vi "Start Functional Test.vi"(5 "New Status of Positions":bool[](array[boolean]), 7 "Rack Number":i16=1 min=1 max=16, 11 "System#":u8=1 min=1 max=16) -> ()   [LabVIEW 2021]
uses:
  Main Controls System v8.0/AutoAge Globals.vi
panel:
  out "At least 1 position\nhas started":bool
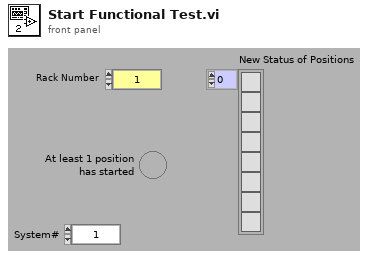
[diagram p1: front panel]
types:
  T1 = enum16{"open", "replace", "create", "open or create", "replace or create", "replace or create with confirmation"}
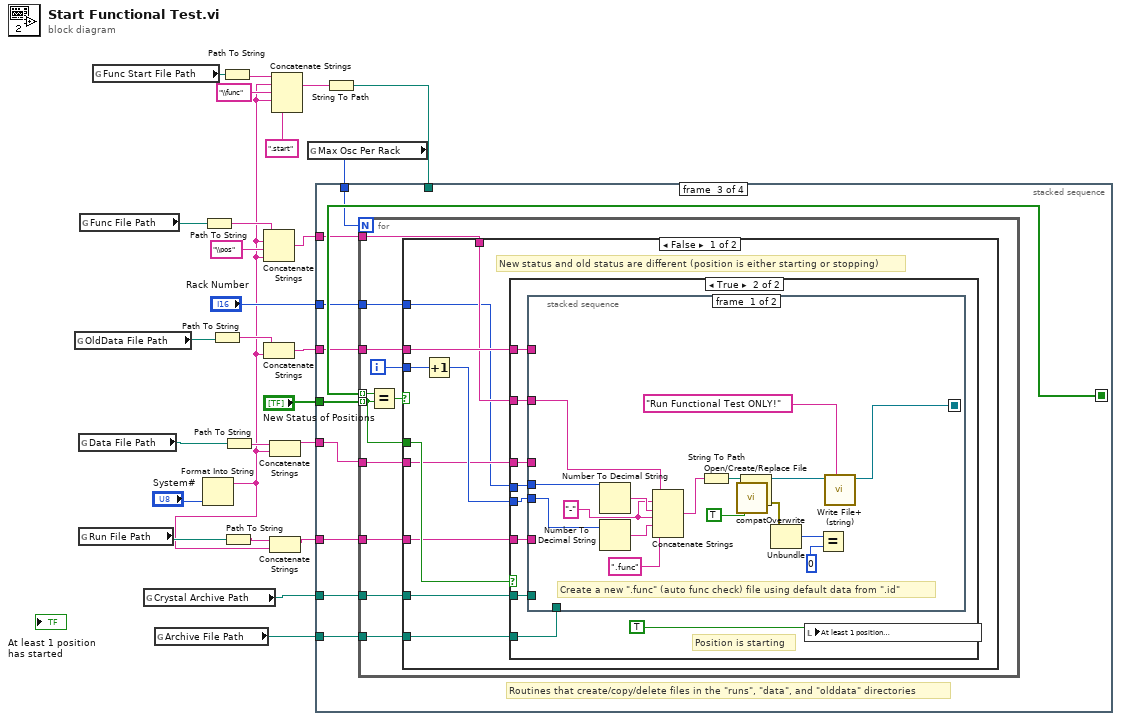
[diagram p0: block diagram]
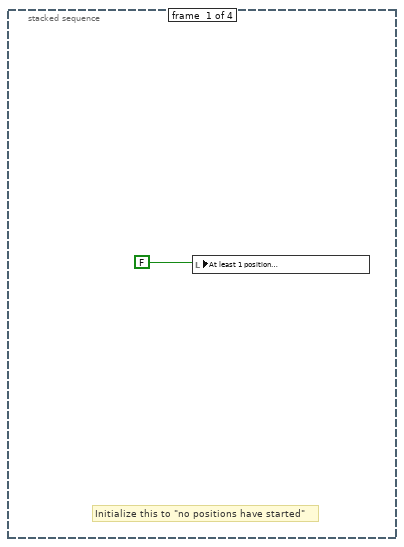
[diagram p2: hidden frame]
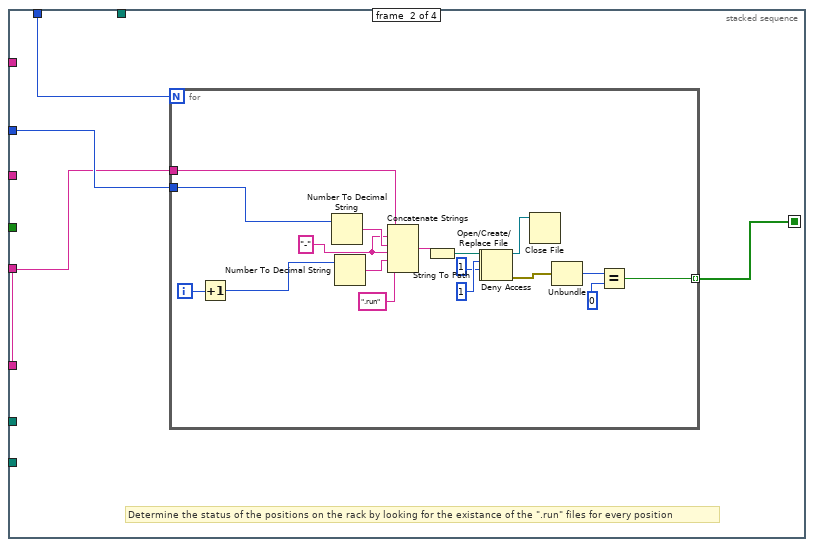
[diagram p3: hidden frame]
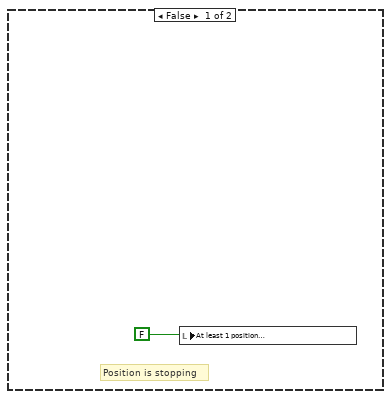
[diagram p4: hidden frame]
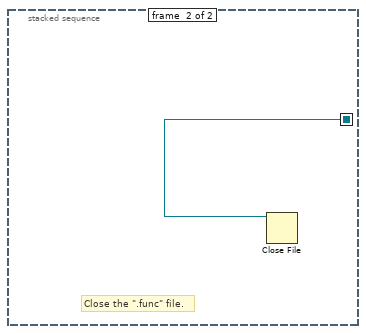
[diagram p5: hidden frame]
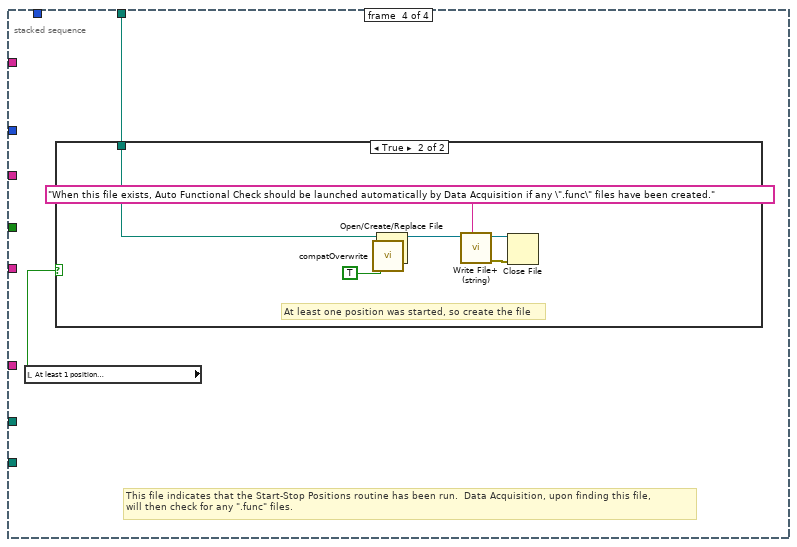
[diagram p7: hidden frame]
diagram:
  n1 = global read "AutoAge Globals.vi" "OldData File Path"() -> (w12:path)
  n2 = global read "AutoAge Globals.vi" "Data File Path"() -> (w11:path)
  n3 = global read "AutoAge Globals.vi" "Run File Path"() -> (w10:path)
  n4 = global read "AutoAge Globals.vi" "Func File Path"() -> (w13:path)
  n5 = global read "AutoAge Globals.vi" "Func Start File Path"() -> (w14:path)
  n6 = global read "AutoAge Globals.vi" "Crystal Archive Path"() -> (w9:path)
  n7 = global read "AutoAge Globals.vi" "Archive File Path"() -> (w8:path)
  n8 = Format Into String("System#") -> (resulting string=w2:string)  [unwired: 3 in, 1 out]
  n9 = Path To String(path=w13) -> (string=w18:string)
  n10 = Path To String(path=w12) -> (string=w20:string)
  n11 = Path To String(path=w14) -> (string=w6:string)
  n12 = Path To String(path=w10) -> (string=w21:string)
  n13 = Path To String(path=w11) -> (string=w24:string)
  n14 = Concatenate Strings(w18, w2, "\\pos" ("Substring"), w2) -> (w17:string)
  n15 = Concatenate Strings(w20, w2) -> (w19:string)
  n16 = Concatenate Strings(w24, w2) -> (w23:string)
  n17 = Concatenate Strings(w21, w2) -> (w22:string)
  n18 = Concatenate Strings(w6, w2, "\\func" ("Substring"), w2, ".start" ("Substring")) -> (w16:string)
  n19 = global read "AutoAge Globals.vi" "Max Osc Per Rack"() -> (w1:u16)
  n20 = String To Path(string=w16) -> (path=w15:path)
  n21 = stacked-sequence {
    seq-local: [_ w30 _ _] -> [_ _ w60 _]
    tunnel: "Rack Number" -> [_ w31 w51 _]
    tunnel: "New Status of Positions" -> [_ _ w59 _]
    tunnel: w22 -> [_ w29 w56 _]
    tunnel: w23 -> [_ _ w57 _]
    tunnel: w19 -> [_ _ w55 _]
    tunnel: w8 -> [_ _ w54 _]
    tunnel: w9 -> [_ _ w53 _]
    tunnel: w17 -> [_ _ w52 _]
    tunnel: w15 -> [_ _ _ w110]
    tunnel: w1 -> [_ w28 w58 _]
    frame #0 {
      # "Initialize this to \"no positions have started\""
      n22 = local write "At least 1 position\nhas started"(FALSE) -> ()
    }
    frame #1 {
      # "Determine the status of the positions on the rack by looking for the existance of the \".run\" files for every position"
      n23 = for {
        N: w28 -> [_]
        tunnel: [w49] -> w30 mode=indexing
        tunnel: w31 -> [w39]
        tunnel: w29 -> [w34]
        i -> [w50]
        w35 = "-"
        n24 = Increment(x=w50) -> (x+1=w36:i32)
        n25 = Number To Decimal String(number=w39) -> (decimal integer string=w38:string)  [unwired: 1 in]
        n26 = Number To Decimal String(number=w36) -> (decimal integer string=w37:string)  [unwired: 1 in]
        n27 = Concatenate Strings(w34, w35, w38, w35, w37, ".run") -> (w48:string)
        n28 = String To Path(string=w48) -> (path=w47:path)
        n29 = Open/Create/Replace File(file path (use dialog)=w47, access (0:read/write)=1) -> (refnum out=w32:refnum<file>, error out=w33:errorcluster)  [unwired: 4 in, 1 out]
        n30 = Deny Access(4:w33, 6:1, 7:w32) -> (0:w44:errorcluster, 3:w41:refnum<file>)
        n31 = Close File(refnum=w41) -> ()  [unwired: 1 in, 2 out]
        n32 = Unbundle(w44) -> ("code"=w42:i32)  [unwired: 2 out]
        n33 = Equal?(x=w42, y=0) -> (x = y?=w49:bool)
      }
    }
    frame #2 {
      # "Routines that create/copy/delete files in the \"runs\", \"data\", and \"olddata\" directories"
      n34 = for {
        N: w58 -> [_]
        tunnel: w60 -> [w70] mode=indexing
        tunnel: w59 -> [w69] mode=indexing
        tunnel: w57 -> [w67]
        tunnel: w56 -> [w66]
        tunnel: w55 -> [w65]
        tunnel: w54 -> [w64]
        tunnel: w53 -> [w63]
        tunnel: w52 -> [w62]
        tunnel: w51 -> [w61]
        i -> [w68]
        n35 = Equal?(x=w70, y=w69) -> (x = y?=w71:bool)
        n36 = case shown="False" w71 {
          tunnel: w69 -> [w81 _]
          tunnel: w68 -> [w80 _]
          tunnel: w67 -> [w78 _]
          tunnel: w66 -> [w77 _]
          tunnel: w65 -> [w76 _]
          tunnel: w64 -> [w75 _]
          tunnel: w63 -> [w74 _]
          tunnel: w62 -> [w73 _]
          tunnel: w61 -> [w72 _]
          frame False {
            # "New status and old status are different (position is either starting or stopping)"
            n37 = Increment(x=w80) -> (x+1=w79:i32)
            n38 = case shown="True" w81 {
              tunnel: w72 -> [_ w83]
              tunnel: w79 -> [_ w91]
              tunnel: w78 -> [_ w89]
              tunnel: w77 -> [_ w85]
              tunnel: w76 -> [_ w88]
              tunnel: w75 -> [_ w87]
              tunnel: w74 -> [_ w86]
              tunnel: w73 -> [_ w84]
              frame False {
                # "Position is stopping"
                n39 = local write "At least 1 position\nhas started"(FALSE) -> ()
              }
              frame True {
                # "Position is starting"
                n40 = stacked-sequence {
                  seq-local: [w96 _] -> [_ w109]
                  tunnel: w83 -> [w97 _]
                  tunnel: w91 -> [w98 _]
                  tunnel: w89 -> [_ _]
                  tunnel: w88 -> [_ _]
                  tunnel: w87 -> [_ _]
                  tunnel: w86 -> [_ _]
                  tunnel: w85 -> [_ _]
                  tunnel: w84 -> [w94 _]
                  frame #0 {
                    w95 = "-"
                    # "Create a new \".func\" (auto func check) file using default data from \".id\""
                    n41 = Number To Decimal String(number=w97) -> (decimal integer string=w101:string)  [unwired: 1 in]
                    n42 = Number To Decimal String(number=w98) -> (decimal integer string=w100:string)  [unwired: 1 in]
                    n43 = Concatenate Strings(w94, w95, w101, w95, w100, ".func") -> (w99:string)
                    n44 = String To Path(string=w99) -> (path=w107:path)
                    n45 = call <vilib>:"compatOverwrite.vi"("overwrite (F)"=TRUE) -> ("overwrite?"=w92:T1)
                    n46 = Open/Create/Replace File(file path (use dialog)=w107, operation (0:open)=w92) -> (refnum out=w103:refnum<file>, error out=w106:errorcluster)  [unwired: 4 in, 1 out]
                    n47 = Unbundle(w106) -> ("code"=w105:i32)  [unwired: 2 out]
                    n48 = Equal?(x=w105, y=0) -> ()  [unwired: 1 out]
                    n49 = call <vilib>:"Write File+ (string).vi"("string"="Run Functional Test ONLY!", "refnum"=w103) -> ("dup refnum"=w96:refnum<file>)  [unwired: 5 in, 2 out]
                  }
                  frame #1 {
                    # "Close the \".func\" file."
                    n50 = Close File(refnum=w109) -> ()  [unwired: 1 in, 2 out]
                  }
                }
                n51 = local write "At least 1 position\nhas started"(TRUE) -> ()
              }
            }
          }
          frame True {
            # "New status and old status are the same, no changes need to be made"
          }
        }
      }
    }
    frame #3 {
      # "This file indicates that the Start-Stop Positions routine has been run.  Data Acquisition, upon finding this file, \nwill then check for any \".func\" files."
      n52 = local read "At least 1 position\nhas started"() -> (w111:bool)
      n53 = case shown="True" w111 {
        tunnel: w110 -> [_ w113]
        frame False {
          # "No positions were started or positions were stopped, so don't create the file"
        }
        frame True {
          # "At least one position was started, so create the file"
          n54 = call <vilib>:"compatOverwrite.vi"("overwrite (F)"=TRUE) -> ("overwrite?"=w112:T1)
          n55 = Open/Create/Replace File(file path (use dialog)=w113, operation (0:open)=w112) -> (refnum out=w115:refnum<file>)  [unwired: 4 in, 2 out]
          n56 = call <vilib>:"Write File+ (string).vi"("string"="When this file exists, Auto Functional Check should be launched automatically by Data Acquisition if any \".func\" files have been created.", "refnum"=w115) -> ("error out"=w117:errorcluster, "dup refnum"=w118:refnum<file>)  [unwired: 5 in, 1 out]
          n57 = Close File(refnum=w118, error in=w117) -> ()  [unwired: 2 out]
        }
      }
    }
  }
